vi "Decompose LabVIEW Object - Interface - Returns No Private Data Clusters.vi"() -> ()   [LabVIEW 2020, in "Composition.Tests.lvlib"]
uses:
  Composition.Tests.lvlib
  IDisposable/IDisposable.lvclass
  <vilib>/addons/_JKI Toolkits/Caraya/classes/Assert/Assert True.vi
  Composition/Composition.lvlib
  <vilib>/addons/_JKI Toolkits/Caraya/classes/Test/Test.lvclass
  <vilib>/addons/_JKI Toolkits/Caraya/classes/Assert/Assert.lvclass
panel:
  out "error out":errorcluster
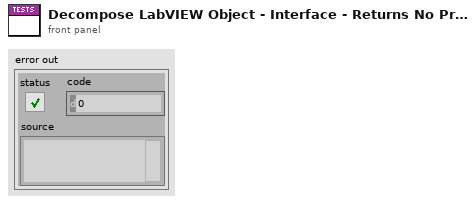
[diagram p1: front panel]
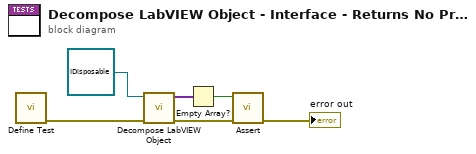
[diagram p0: block diagram]
diagram:
  n1 = call <vilib>:"Define Test.vi"() -> ("error out"=w4:errorcluster)  [unwired: 11 in]
  n2 = call "Decompose LabVIEW Object.vi"("error in (no error)"=w4, "LabVIEW Object"=refnum<class "IDisposable.lvclass"> refnum ("Reflection.Tests.lvlib:String.lvclass")) -> ("error out"=w3:errorcluster, "Private Data Clusters"=w2:variant[])  [unwired: 6 in, 2 out]
  n3 = Empty Array?(array=w2) -> (empty?=w1:bool)
  n4 = call-poly <vilib>:"Assert.vi"("error in (no error)"=w3, "True?"=w1) -> ("error out"=→"error out":errorcluster)  [unwired: 9 in]
